vi "Sub.vi"(3 "上取整(F)":bool, 4 "最大值":i64=100) -> (1 "随机生成的整数":i64=56)   [LabVIEW 2016]
panel:
  out "浮点数":dbl=55.066686853691536
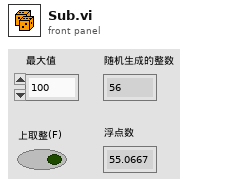
[diagram p1: front panel]
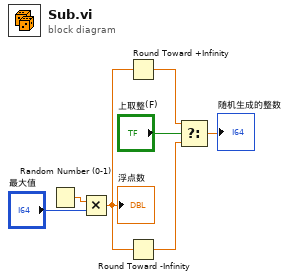
[diagram p0: block diagram]
diagram:
  n1 = Random Number (0-1)() -> (number: 0 to 1=w7:dbl)
  n2 = Multiply(x=w7, y="最大值") -> (x*y=w4:dbl)
  "浮点数" <- w4
  n3 = Round Toward +Infinity(x=w4) -> (ceil(x): smallest int >= x=w5:dbl)
  n4 = Round Toward -Infinity(1:w4) -> (0:w2:dbl)
  n5 = Select(t=w5, s="上取整(F)", f=w2) -> (s? t:f=→"随机生成的整数":dbl)
